vi "Configure Basic Histogram.vi"(5 "Exponential Fit (T: Enable)":bool=TRUE, 6 "Number Of Histogram Bins (0: hb16)":i32(ring) items=["hb16", "hb32", "hb64", "hb128", "hb256", "hb512"], 7 "Sample Size (0: hs64k)":i32(ring) items=["hs64k", "hs32k", "hs16k", "hs8k", "hs4k", "hs2k", "hs1k", "hs512"], 8 "error in (no error)":errorcluster, 9 "Sampling Frequency Divider (0: hdFsdiv1)":i32(ring) items=["hdFsdiv1", "hdFsdiv2", "hdFsdiv4", "hdFsdiv8", "hdFsdiv16", "hdFsdiv32", "hdFsdiv64", "hdFsdiv128", "hdFsdiv256", "hdFsdiv512"], 10 "Analyzer (0: A0)":i32(ring) items=["A0", "A1"], 11 "VISA resource name":refnum<visa-resource-name>) -> (0 "error out":errorcluster, 3 "VISA resource name out":refnum<visa-resource-name>)   [LabVIEW 2014, in "Stanford Research SR1.lvlib"]
doc: "Configures the basic attributes for the Histogram Analyzer."
uses:
  Stanford Research SR1.lvlib
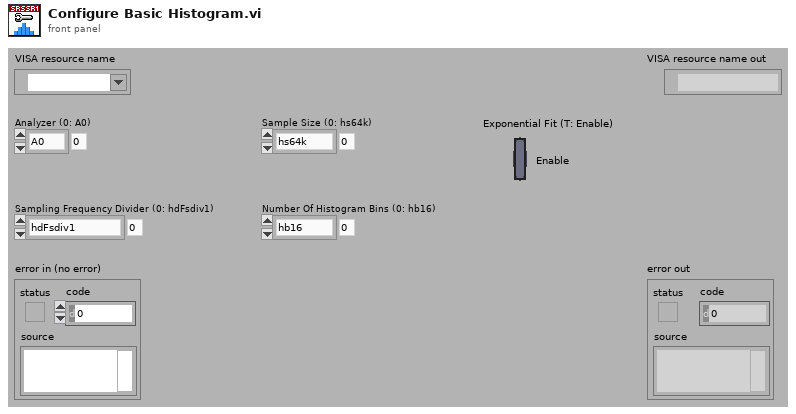
[diagram p1: front panel]
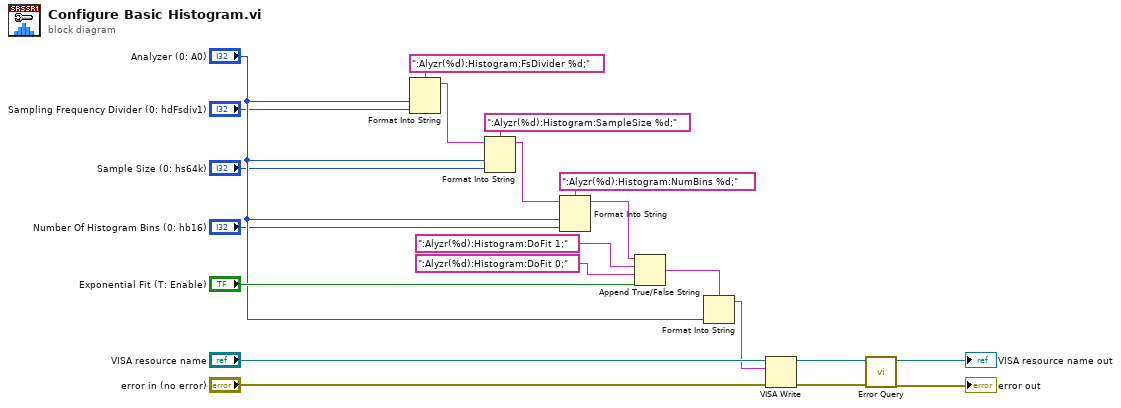
[diagram p0: block diagram]
diagram:
  n1 = Format Into String(format string=":Alyzr(%d):Histogram:FsDivider %d;", "Analyzer (0: A0)", "Sampling Frequency Divider (0: hdFsdiv1)") -> (resulting string=w20:string)  [unwired: 2 in, 1 out]
  n2 = Format Into String(format string=":Alyzr(%d):Histogram:SampleSize %d;", initial string=w20, "Analyzer (0: A0)", "Sample Size (0: hs64k)") -> (resulting string=w18:string)  [unwired: 1 in, 1 out]
  n3 = Format Into String(format string=":Alyzr(%d):Histogram:NumBins %d;", initial string=w18, "Analyzer (0: A0)", "Number Of Histogram Bins (0: hb16)") -> (resulting string=w16:string)  [unwired: 1 in, 1 out]
  n4 = Append True/False String(1:"Exponential Fit (T: Enable)", 2:":Alyzr(%d):Histogram:DoFit 0;", 3:":Alyzr(%d):Histogram:DoFit 1;", 4:w16) -> (0:w6:string)
  n5 = Format Into String(format string=w6, "Analyzer (0: A0)") -> (resulting string=w1:string)  [unwired: 2 in, 1 out]
  n6 = VISA Write(VISA resource name="VISA resource name", write buffer=w1, error in (no error)="error in (no error)") -> (VISA resource name out=w10:refnum<visa-resource-name>, error out=w9:errorcluster)  [unwired: 1 out]
  n7 = call "Error Query.vi"("error in (no error)"=w9, "VISA resource name"=w10) -> ("error out"=→"error out":errorcluster, "VISA resource name out"=→"VISA resource name out":refnum<visa-resource-name>)  [unwired: 6 in, 2 out]
